vi "Write Nodes.vi"(8 "error in (no error)":errorcluster, 10 "Nodes":refnum<class "abs_Node.lvclass">[](array[class]), 11 "abs_Composite in":refnum<class "abs_Composite.lvclass">) -> (0 "error out":errorcluster, 3 "abs_Composite out":refnum<class "abs_Composite.lvclass">)   [LabVIEW 2021, in "BT.lvlib" / "abs_Composite.lvclass"]
uses:
  abs_Composite.lvclass
  abs_Node/abs_Node.lvclass
  abs_Composite.lvclass/abs_Composite.ctl
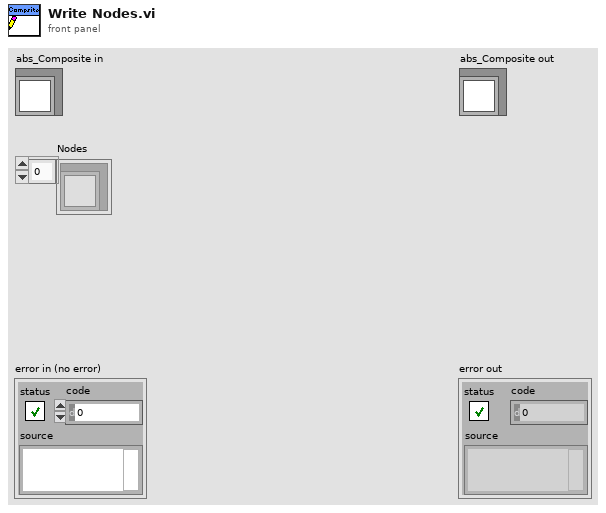
[diagram p1: front panel]
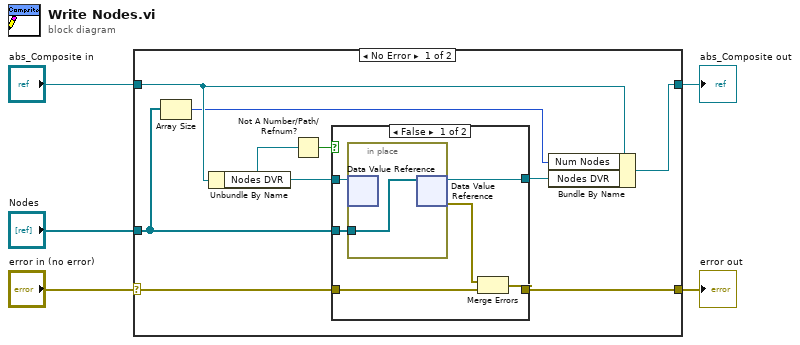
[diagram p0: block diagram]
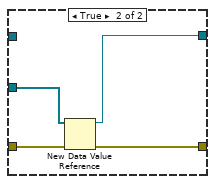
[diagram p2: hidden frame]
diagram:
  n1 = case shown="No Error" "error in (no error)" {
    selector: "error in (no error)" -> [w12 w26]
    tunnel: [w10 w26] -> w4
    tunnel: [w14 w27] -> w2
    tunnel: "abs_Composite in" -> [w13 w27]
    tunnel: "Nodes" -> [w7 _]
    frame No Error {
      n2 = Array Size(array=w7) -> (size(s)=w6:i32)
      n3 = Unbundle By Name(w13) -> ("Nodes DVR"=w8:refnum<data-value>)
      n4 = Not A Number/Path/Refnum?(number/path/refnum=w8) -> (NaN/Path/Refnum?=w9:bool)
      n5 = case shown="False" w9 {
        tunnel: w12 -> [w20 w25]
        tunnel: w7 -> [w17 w24]
        tunnel: [w18 w23] -> w11
        tunnel: [w16 w22] -> w10
        tunnel: w8 -> [w19 _]
        frame False {
          n6 = in-place {
            in-place-border: w17 -> [w21]
            n7 = in-place-dvr #1(w19) -> ()  [unwired: 2 out]
            n8 = in-place-dvr #1(w21) -> (w18:refnum<data-value>, w15:errorcluster)
          }
          n9 = Merge Errors(w15, w20) -> (w16:errorcluster)
        }
        frame True {
          n10 = New Data Value Reference(data value=w24, error in=w25) -> (data value reference=w23:refnum<data-value>, error out=w22:errorcluster)
        }
      }
      n11 = Bundle By Name(cluster=w13, "Num Nodes"=w6, "Nodes DVR"=w11) -> (w14:refnum<class "abs_Composite.lvclass">)
    }
    frame Error {
    }
  }
  "error out" <- w4
  "abs_Composite out" <- w2
